vi "Background Config File Update.vi"   [LabVIEW 2014]
uses:
  Robot Global Data.vi
  GlobalConfig.vi
types:
  T1 = typedef "WPI_DriverStationRobotMode2.ctl" = enum16{"Autonomous Disabled", "Autonomous Enabled", "Teleop Disabled", "Teleop Enabled", "Disconnected", "Finish", "Test Disabled", "Test Enabled", "Emergency Stopped"}
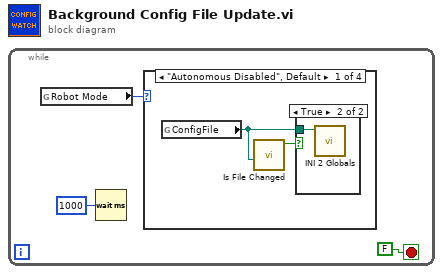
[diagram p0: block diagram]
diagram:
  n1 = while {
    stop <- FALSE stop-if-true
    n2 = global read "Robot Global Data.vi" "Robot Mode"() -> (w2:T1)
    n3 = Wait (ms)(milliseconds to wait=u32 1000) -> ()  [unwired: 1 out]
    n4 = case shown="\"Autonomous Disabled\", Default" w2 {
      frame "Autonomous Disabled", Default {
        n5 = global read "GlobalConfig.vi" "ConfigFile"() -> (w4:path)
        n6 = call "Is File Changed.vi"("path"=w4) -> ("Changed"=w5:bool)  [unwired: 9 in]
        n7 = case shown="True" w5 {
          tunnel: w4 -> [_ w6]
          frame False {
          }
          frame True {
            n8 = call "INI 2 Globals.vi"("configuration file path"=w6) -> ()  [unwired: 10 in, 1 out]
          }
        }
      }
      frame "Autonomous Enabled" {
      }
      frame "Teleop Enabled" {
      }
      frame "Test Enabled" {
      }
    }
  }
